vi "AgentConfigTester.vi"() -> ()   [LabVIEW 2013]
uses:
  FA_NativeTypes API/source/VI Source/FA_Config.ctl
  FA_LocalStore API/source/VI Source/FA_LSSpecialTypes.ctl
  FA_AgentConfig.ctl
  FA_LocalStore API/source/VI Source/FA_LocalStore.lvlib
  FA_AgentConfig.lvlib
  FA_NativeTypes API/source/VI Source/FA_NativeTypes.lvlib
panel:
  out "Error Out":errorcluster
  out "DebugStatus":bool
  out "CloudLookupTime":u32
  out "Config":T1
  out "AgentConfig":T3
  out "ConfigData":T1
  out "XML String":string
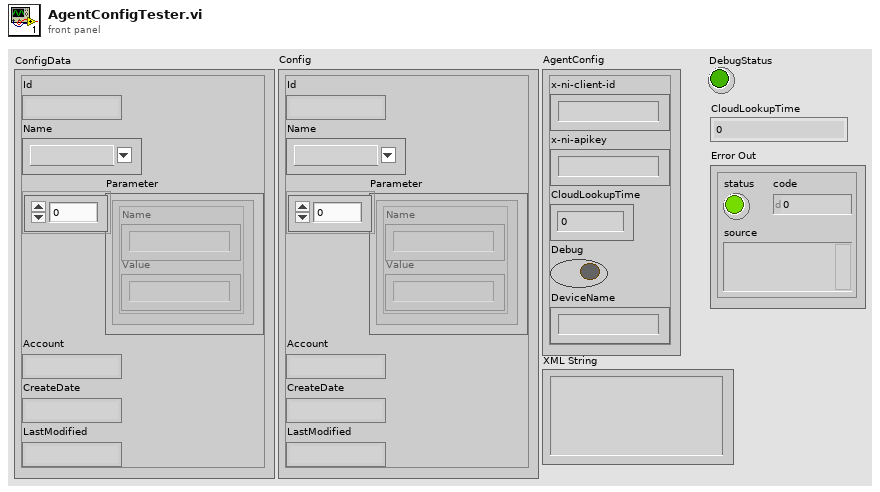
[diagram p1: front panel]
types:
  T1 = typedef "FA_NativeTypes.lvlib/FA_Config.ctl" = cluster{"Id":string, "Name":T2, "Parameter":cluster{"Name":string, "Value":string}[], "Account":string, "CreateDate":string, "LastModified":string}
  T2 = typedef "FA_LocalStore.lvlib/FA_LSSpecialTypes.ctl" = string
  T3 = typedef "FA_AgentConfig.lvlib/FA_AgentConfig.ctl" = cluster{"x-ni-client-id":string, "x-ni-apikey":string, "CloudLookupTime":u32, "Debug":bool, "DeviceName":string}
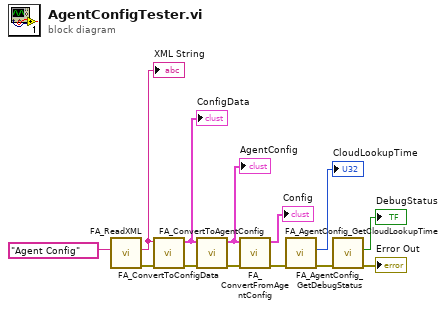
[diagram p0: block diagram]
diagram:
  n1 = call "FA_ReadXML.vi"("Special Type"=T2 "Agent Config") -> ("Error Out"=w7:errorcluster, "XML String"=w12:string)  [unwired: 7 in]
  "XML String" <- w12
  n2 = call "FA_ConvertToConfigData.vi"("Error In"=w7, "XML String"=w12) -> ("Error Out"=w8:errorcluster, "ConfigData"=w11:T1)  [unwired: 8 in]
  "ConfigData" <- w11
  n3 = call "FA_ConvertToAgentConfig.vi"("Error In"=w8, "Config"=w11) -> ("Error Out"=w9:errorcluster, "AgentConfig"=w10:T3)  [unwired: 8 in]
  "AgentConfig" <- w10
  n4 = call "FA_ConvertFromAgentConfig.vi"("Error In"=w9, "AgentConfig"=w10) -> ("Error Out"=w5:errorcluster, "Config"=→"Config":T1)  [unwired: 8 in]
  n5 = call "FA_AgentConfig_GetCloudLookupTime.vi"("Error In"=w5) -> ("Error Out"=w3:errorcluster, "CloudLookupTime"=→"CloudLookupTime":u32)  [unwired: 9 in]
  n6 = call "FA_AgentConfig_GetDebugStatus.vi"("Error In"=w3) -> ("Error Out"=→"Error Out":errorcluster, "DebugStatus"=→"DebugStatus":bool)  [unwired: 9 in]
